vi "Continuous Stimuli Test.vi"() -> ()   [LabVIEW 2015]
uses:
  <vilib>/sound2/lvsound2.llb/Sampling Mode.ctl
  <vilib>/sound2/lvsound2.llb/Sound Data Format.ctl
  Waveform VIs/Tone VIs/Tone Params.ctl
  <vilib>/sound2/lvsound2.llb/Sound Output Write (DBL Single).vi
panel:
  in  "Slide":dbl(slide)=100.0 min=100.0 max=600.0 step=1.0 scale=100.0..600.0
  in  "Sampling Rate (Hz)":dbl=20000.0
  out "Time":dbl[](graph)
  in  "Stop":bool
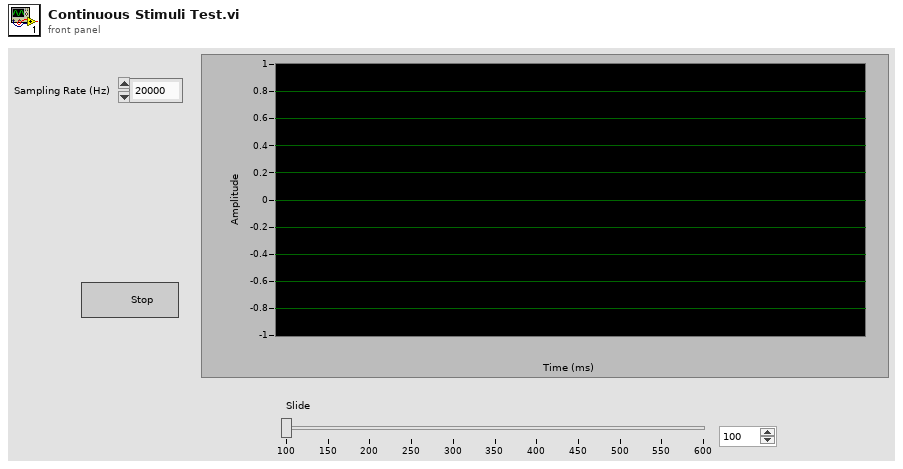
[diagram p1: front panel]
types:
  T1 = typedef "Tone Params.ctl" = cluster{"Frequency (kHz)":dbl, "Last Freq":dbl, "Last Phase":dbl}
  T2 = typedef "Sound Data Format.ctl" = cluster{"sample rate (S/s)":dbl, "number of channels":i32, "bits per sample":i32}
  T3 = typedef "Sampling Mode.ctl" = i32
  T4 = typedef "Sound Output Task ID.ctl" = u32
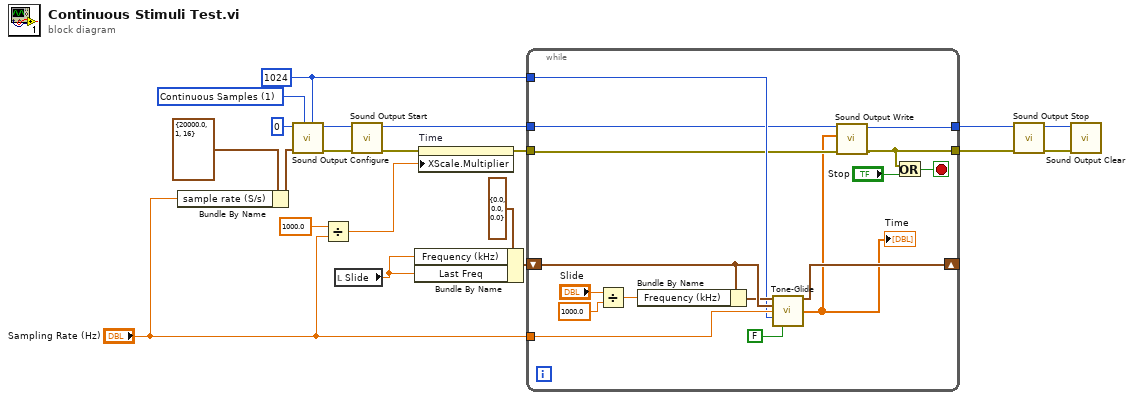
[diagram p0: block diagram]
diagram:
  w5 = 1024 ("number of samples/ch")
  w19 = T3 1 items=["Finite Samples", "Continuous Samples"] ("sample mode")
  n1 = Bundle By Name(cluster=T2 {"sample rate (S/s)"=20000.0, "number of channels"=1, "bits per sample"=16} ("sound format"), "sample rate (S/s)"="Sampling Rate (Hz)") -> (w8:T2)
  n2 = call <vilib>:"Sound Output Configure.vi"("number of samples/ch"=w5, "sample mode"=w19, "sound format"=w8, "device ID"=u32 0) -> ("error out"=w17:errorcluster, "task ID"=w16:T4)  [unwired: 6 in]
  n3 = Divide(x=1000.0, y="Sampling Rate (Hz)") -> (x/y=w6:dbl)
  n4 = local read "Slide"() -> (w2:dbl)
  n5 = call <vilib>:"Sound Output Start.vi"("error in (no error)"=w17, "task ID"=w16) -> ("error out"=w10:errorcluster, "task ID out"=w15:T4)  [unwired: 8 in]
  n6 = Bundle By Name(cluster=T1 {"Frequency (kHz)"=0.0, "Last Freq"=0.0, "Last Phase"=0.0} ("Old"), "Frequency (kHz)"=w2, "Last Freq"=w2) -> (w3:T1)
  n7 = property on="Time" class="WFGraph (strict)"(error in=w10, "XScale.Multiplier"=w6) -> (error out=w9:errorcluster)  [unwired: 1 in, 1 out]
  n8 = while {
    tunnel: w9 -> [w23]
    tunnel: w15 -> [w26]
    tunnel: [w24] -> w14
    tunnel: [w25] -> w13
    tunnel: w5 -> [w29]
    shift-right: [w31] -> _
    shift-left: w3 -> [w33]
    tunnel: "Sampling Rate (Hz)" -> [w30]
    stop <- w35 stop-if-true
    n9 = Divide(x="Slide", y=1000.0) -> (x/y=w28:dbl)
    n10 = Bundle By Name(cluster=w33, "Frequency (kHz)"=w28) -> (w32:T1)
    n11 = call "Tone-Glide.vi"("New"=w32, "Old"=w33, "Fs (Hz)"=w30, "Npts"=w29, "Original method?"=FALSE) -> ("Params out"=w31:T1, "Y"=w22:dbl[])  [unwired: 9 in]
    "Time" <- w22
    n12 = call-poly <vilib>:"Sound Output Write.vi"("error in (no error)"=w23, "data"=w22, "task ID"=w26) -> ("error out"=w24:errorcluster, "task ID out"=w25:T4)  [unwired: 7 in]
    n13 = Or(x=w24, y="Stop") -> (x .or. y?=w35:bool)
  }
  n14 = call <vilib>:"Sound Output Stop.vi"("error in (no error)"=w14, "task ID"=w13) -> ("error out"=w12:errorcluster, "task ID out"=w11:T4)  [unwired: 8 in]
  n15 = call <vilib>:"Sound Output Clear.vi"("error in (no error)"=w12, "task ID"=w11) -> ()  [unwired: 9 in, 1 out]
